vi "Step Update.vi"(8 "error in (no error)":errorcluster, 10 "Step Record (empty)":T2, 11 "Connection Refnum":T1) -> (0 "error out":errorcluster, 3 "Connection Refnum":T1)   [LabVIEW 2011]
uses:
  Step Record.ctl
  SI.LIB/ODBC/SQL Controls/Connection Refnum.ctl
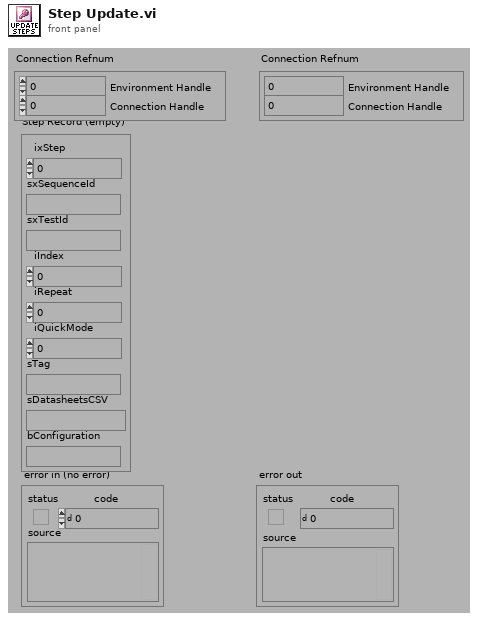
[diagram p1: front panel]
types:
  T1 = typedef "Connection Refnum.ctl" = cluster{"Environment Handle":i32, "Connection Handle":i32}
  T2 = typedef "Step Record.ctl" = cluster{"ixStep":i32, "sxSequenceId":string, "sxTestId":string, "iIndex":i32, "iRepeat":i32, "iQuickMode":i32, "sTag":string, "sDatasheetsCSV":string, "bConfiguration":string}
  T3 = typedef "Statement Refnum.ctl" = cluster{"Statement Handle":i32, "Parameter Number":u16}
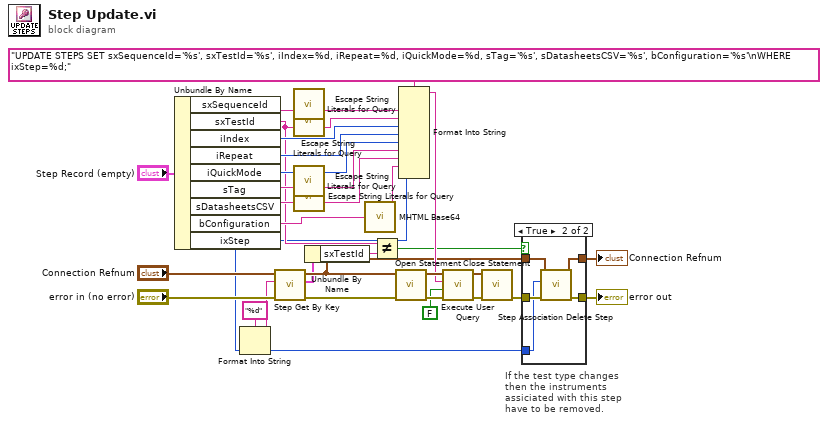
[diagram p0: block diagram]
diagram:
  # "If the test type changes\nthen the instruments\nassiciated with this step\nhave to be removed."
  n1 = Unbundle By Name("Step Record (empty)") -> ("sxSequenceId"=w26:string, "sxTestId"=w3:string, "iIndex"=w23:i32, "iRepeat"=w22:i32, "iQuickMode"=w21:i32, "sTag"=w20:string, "sDatasheetsCSV"=w18:string, "bConfiguration"=w16:string, "ixStep"=w1:i32)
  n2 = Format Into String(format string="%d", w1) -> (resulting string=w10:string)  [unwired: 2 in, 1 out]
  n3 = call "Step Get By Key.vi"("error in (no error)"="error in (no error)", "ixStep"=w10, "Connection Refnum"="Connection Refnum") -> ("error out"=w12:errorcluster, "Step Record"=w5:T2, "Connection Refnum"=w9:T1)  [unwired: 5 in, 1 out]
  n4 = call "Escape String Literals for Query.vi"("String"=w26) -> ("escaped String"=w25:string)  [unwired: 1 in, 13 out]
  n5 = call "Escape String Literals for Query.vi"("String"=w3) -> ("escaped String"=w24:string)  [unwired: 1 in, 13 out]
  n6 = call "Escape String Literals for Query.vi"("String"=w20) -> ("escaped String"=w19:string)  [unwired: 1 in, 13 out]
  n7 = call "Escape String Literals for Query.vi"("String"=w18) -> ("escaped String"=w17:string)  [unwired: 1 in, 13 out]
  n8 = Unbundle By Name(w5) -> ("sxTestId"=w4:string)
  n9 = call "MHTML Base64.vi"("Binary String"=w16) -> ("String (Base64)"=w15:string)  [unwired: 14 out]
  n10 = Not Equal?(x=w3, y=w4) -> (x != y?=w2:bool)
  n11 = call "Open Statement.vi"("error in (no error)"=w12, "Connection Refnum"=w9) -> ("error out"=w32:errorcluster, "Statement Refnum"=w31:T3)  [unwired: 4 out]
  n12 = Format Into String(format string="UPDATE STEPS SET sxSequenceId='%s', sxTestId='%s', iIndex=%d, iRepeat=%d, iQuickMode=%d, sTag='%s', sDatasheetsCSV='%s', bConfiguration='%s'\nWHERE ixStep=%d;" ("User Query"), w25, w24, w23, w22, w21, w19, w17, w15, w1) -> (resulting string=w29:string)  [unwired: 2 in, 1 out]
  n13 = call "Execute User Query.vi"("error in (no error)"=w32, "Return Data? (f)"=FALSE, "User Query"=w29, "Statement Refnum"=w31) -> ("error out"=w33:errorcluster, "Statement Refnum"=w34:T3)  [unwired: 2 out]
  n14 = call "Close Statement.vi"("error in (no error)"=w33, "Statement Refnum"=w34) -> ("error out"=w8:errorcluster)  [unwired: 5 out]
  n15 = case shown="True" w2 {
    tunnel: w9 -> [w36 w38]
    tunnel: w8 -> [w35 w41]
    tunnel: [w36 w39] -> w7
    tunnel: [w35 w40] -> w6
    tunnel: w1 -> [_ w37]
    frame False {
    }
    frame True {
      n16 = call "Step Association Delete Step.vi"("error in (no error)"=w41, "iStep (0)"=w37, "Connection Refnum"=w38) -> ("error out"=w40:errorcluster, "Connection Refnum"=w39:T1)  [unwired: 7 in]
    }
  }
  "error out" <- w6
  "Connection Refnum" <- w7
